vi "Measure.vi"(7 "Sporks Number":i32, 8 "error in":errorcluster, 11 "VISA resource in":refnum<visa-resource-name>) -> (0 "error out":errorcluster, 1 "Spork":i32[](array[numeric]), 2 "Deviation":i32[](array[numeric]), 3 "VISA resource out":refnum<visa-resource-name>, 6 "Timeout":bool)   [LabVIEW 2025]
uses:
  <vilib>/Utility/error.llb/Trim Whitespace One-Sided.vi
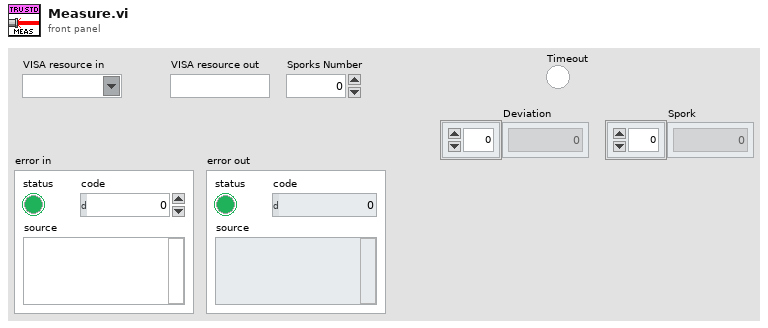
[diagram p1: front panel]
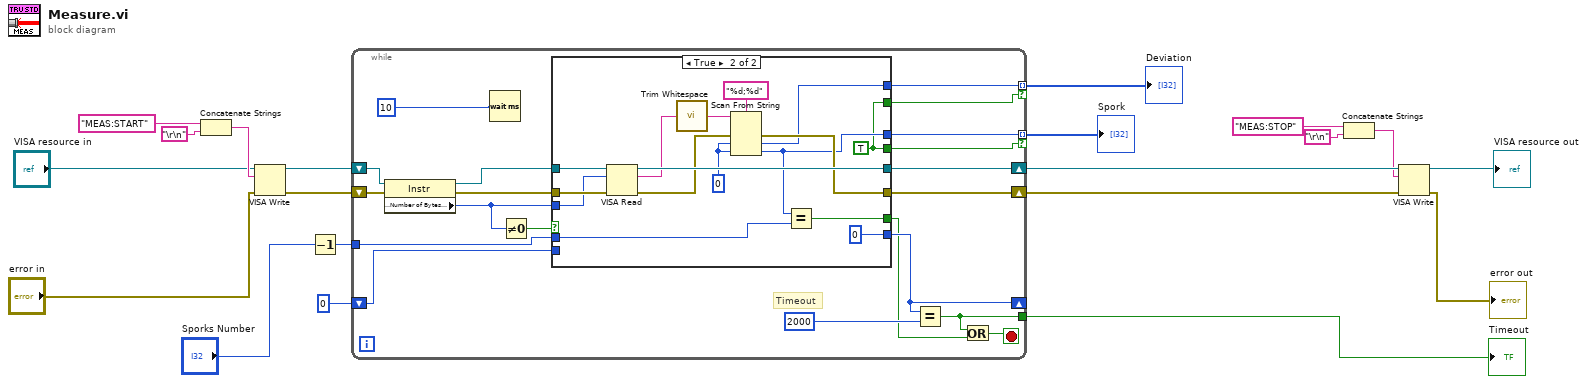
[diagram p0: block diagram]
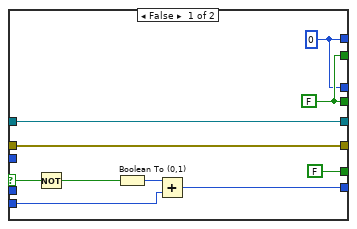
[diagram p2: hidden frame]
diagram:
  n1 = Concatenate Strings("MEAS:START" ("string"), "\r\n") -> (w20:string)
  n2 = VISA Write(VISA resource name="VISA resource in", write buffer=w20, error in (no error)="error in") -> (VISA resource name out=w17:refnum<visa-resource-name>, error out=w16:errorcluster)  [unwired: 1 out]
  n3 = Decrement(x="Sporks Number") -> (x-1=w2:i32)
  n4 = while {
    shift-right: [w36] -> w13
    shift-left: w17 -> [w38]
    shift-right: [w37] -> w12
    shift-left: w16 -> [w35]
    shift-right: [w29] -> _
    shift-left: i16 0 -> [w30]
    tunnel: [w27] -> w5
    tunnel: w2 -> [w26]
    tunnel: [w24] -> w4 mode=indexing if=w22
    tunnel: [w23] -> w3 mode=indexing if=w21
    stop <- w28 stop-if-true
    # "Timeout"
    n5 = property class="Instr"(reference=w38, error in=w35) -> (reference out=w40:refnum<visa-resource-name>, error out=w39:errorcluster, "Serial Settings:Number of Bytes at Serial Port"=w33:u32)
    n6 = Wait (ms)(milliseconds to wait=u32 10) -> ()  [unwired: 1 out]
    n7 = Not Equal To 0?(x=w33) -> (x != 0?=w32:bool)
    n8 = case shown="True" w32 {
      selector: w32 -> [w48 _]
      tunnel: w40 -> [w50 w66]
      tunnel: w39 -> [w49 w65]
      tunnel: [w49 w60] -> w37
      tunnel: [w50 w64] -> w36
      tunnel: w33 -> [_ w63]
      tunnel: w30 -> [w45 _]
      tunnel: [w44 i16 0] -> w29
      tunnel: w26 -> [_ w55]
      tunnel: [FALSE w54] -> w25
      tunnel: [w41 w52] -> w24
      tunnel: [w41 w53] -> w23
      tunnel: [w42 w51] -> w22
      tunnel: [w42 w51] -> w21
      frame False {
        w41 = 0 ("default value 14")
        w42 = FALSE
        n9 = Not(x=w48) -> (.not. x?=w47:bool)
        n10 = Boolean To (0,1)(Boolean=w47) -> (0, 1=w46:i16)
        n11 = Add(x=w46, y=w45) -> (x+y=w44:i16)
      }
      frame True {
        w51 = TRUE
        w56 = 0 ("default value 14")
        n12 = VISA Read(VISA resource name=w66, byte count=w63, error in (no error)=w65) -> (VISA resource name out=w64:refnum<visa-resource-name>, read buffer=w57:string, error out=w61:errorcluster)  [unwired: 1 out]
        n13 = call <vilib>:"Trim Whitespace.vi"("string"=w57) -> ("trimmed string"=w58:string)  [unwired: 1 in]
        n14 = Scan From String(format string="%d;%d", input string=w58, error in=w61, default 1=w56, default 2=w56) -> (error out=w60:errorcluster, output 1=w53:i32, output 2=w52:i32)  [unwired: 1 in, 2 out]
        n15 = Equal?(x=w52, y=w55) -> (x = y?=w54:bool)
      }
    }
    n16 = Equal?(x=w29, y=i16 2000) -> (x = y?=w27:bool)
    n17 = Or(x=w27, y=w25) -> (x .or. y?=w28:bool)
  }
  "Timeout" <- w5
  "Spork" <- w4
  "Deviation" <- w3
  n18 = Concatenate Strings("MEAS:STOP" ("string"), "\r\n") -> (w11:string)
  n19 = VISA Write(VISA resource name=w13, write buffer=w11, error in (no error)=w12) -> (VISA resource name out=→"VISA resource out":refnum<visa-resource-name>, error out=→"error out":errorcluster)  [unwired: 1 out]
